vi "EX_Open232.vi"(8 "error in (no error)":errorcluster, 10 "baud rate (9600)":u32=9600, 11 "VISA resource name":refnum<visa-resource-name>) -> (0 "error out":errorcluster, 3 "status":bool)   [LabVIEW 2017]
uses:
  <vilib>/Instr/_visa.llb/VISA Configure Serial Port (Instr).vi
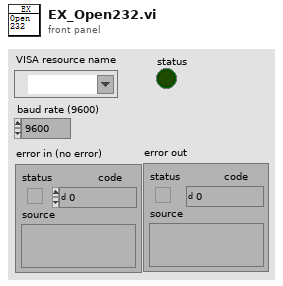
[diagram p1: front panel]
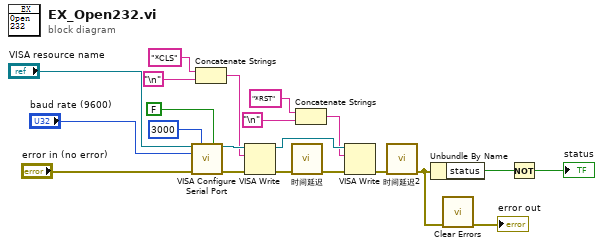
[diagram p0: block diagram]
diagram:
  n1 = call-poly "VISA Configure Serial Port"("VISA resource name"="VISA resource name", "timeout (10sec)"=u32 3000, "Enable Termination\nChar (T)"=FALSE ("Enable Termination\nChar (T)"), "baud rate (9600)"="baud rate (9600)", "error in (no error)"="error in (no error)") -> ("VISA resource name out"=w12:refnum<visa-resource-name>, "error out"=w18:errorcluster)  [unwired: 9 in]
  n2 = Concatenate Strings("*CLS" ("写入缓冲区"), "\n") -> (w6:string)
  n3 = VISA Write(VISA resource name=w12, write buffer=w6, error in (no error)=w18) -> (VISA resource name out=w9:refnum<visa-resource-name>, error out=w7:errorcluster)  [unwired: 1 out]
  n4 = call "时间延迟"("error in (no error)"=w7) -> ("error out"=w4:errorcluster)  [unwired: 10 in]
  n5 = Concatenate Strings("*RST" ("写入缓冲区"), "\n") -> (w8:string)
  n6 = VISA Write(VISA resource name=w9, write buffer=w8, error in (no error)=w4) -> (error out=w11:errorcluster)  [unwired: 2 out]
  n7 = call "时间延迟2"("error in (no error)"=w11) -> ("error out"=w3:errorcluster)  [unwired: 10 in]
  n8 = Unbundle By Name(w3) -> ("status"=w16:bool)
  n9 = call <vilib>:"Clear Errors.vi"("error in (no error)"=w3) -> ("error out"=→"error out":errorcluster)  [unwired: 5 in, 1 out]
  n10 = Not(x=w16) -> (.not. x?=→"status":bool)
